vi "Find Param Array Length (SubVI).vi"(11 "JSON String":string) -> (0 "Variable Array":string[](array[string]), 1 "Token Array":T1[](array[typedef]), 2 "Length":i32, 3 "Index":i32)   [LabVIEW 2013]
uses:
  Library/Token.ctl
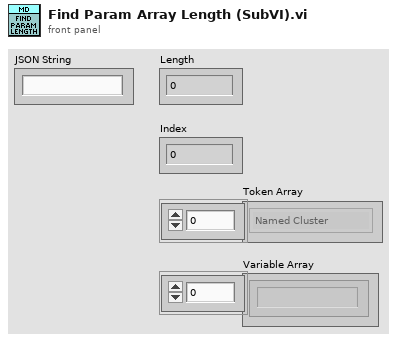
[diagram p1: front panel]
types:
  T1 = typedef "Token.ctl" = enum16{"End", "Boolean", "Named Cluster", "Unnamed Cluster", "Array", "String", "Decimal", "FloatingPoint", "End Array", "End Cluster"}
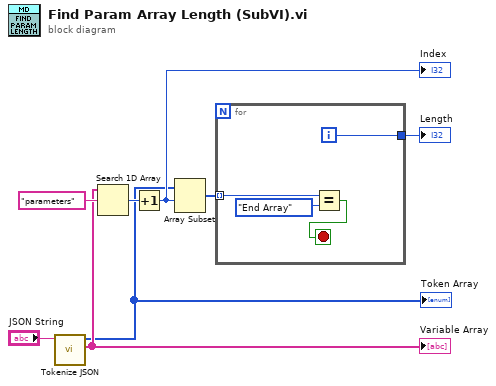
[diagram p0: block diagram]
diagram:
  n1 = call "Tokenize JSON.vi"("JSON String"="JSON String") -> ("Variable Names"=w2:string[], "Token Array"=w1:T1[])  [unwired: 9 in]
  "Variable Array" <- w2
  "Token Array" <- w1
  n2 = Search 1D Array(1D array=w2, element="parameters" ("y")) -> (index of element=w5:i32)  [unwired: 1 in]
  n3 = Increment(x=w5) -> (x+1=w6:i32)
  "Index" <- w6
  n4 = Array Subset(array=w1, index=w6) -> (w7:T1[])  [unwired: 1 in]
  n5 = for {
    tunnel: w7 -> [w12] mode=indexing
    tunnel: [w9] -> w8
    i -> [w9]
    stop <- w10 stop-if-true
    n6 = Equal?(x=w12, y=Token."End Array") -> (x = y?=w10:bool)
  }
  "Length" <- w8
